vi "scanallvalues.vi"(0 "VISA resource name out":refnum<visa-resource-name>, 1 "nm ch":i32[](array[numeric]), 2 "Voltages values":dbl[](array[numeric]), 3 "Init clip value":i32[](array[numeric]), 4 "base path":path, 5 "error in":errorcluster, 6 "Integration Board IP":string, 7 "L1 Address":i32, 8 "Save test data":bool=TRUE, 9 "Ch burst":i32, 11 "Init att value":i32[](array[numeric])) -> (14 "50%":dbl[][][][](array[numeric]), 15 "L1 min values":i32[](array[numeric])=[180, 378, 779, 1613, 2478, 4286, 5228, 6743], 19 "error out":errorcluster)   [LabVIEW 2009]
uses:
  <instrlib>/Agilent 81150/Agilent 81150.lvlib
  <vilib>/Analysis/NI_AALPro.lvlib
panel:
  out "Data out":string="ACK\r\n"
  out "XY Graph":cluster{"Y":dbl[], "Y":dbl[]}[](graph)
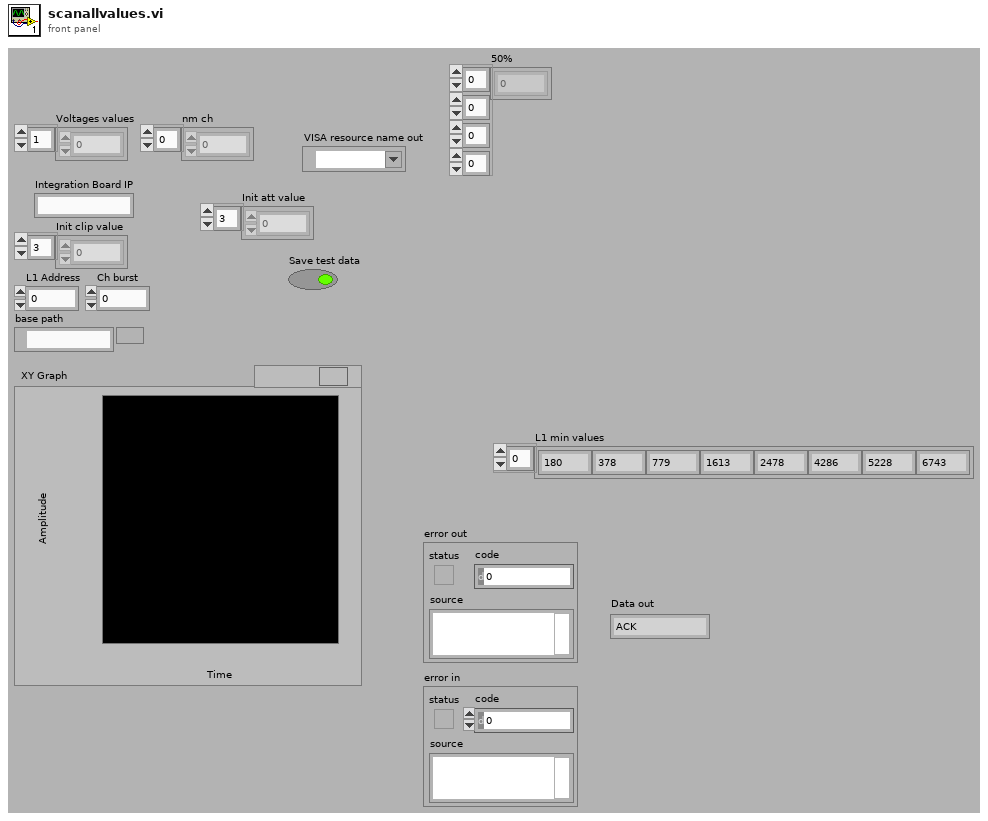
[diagram p1: front panel]
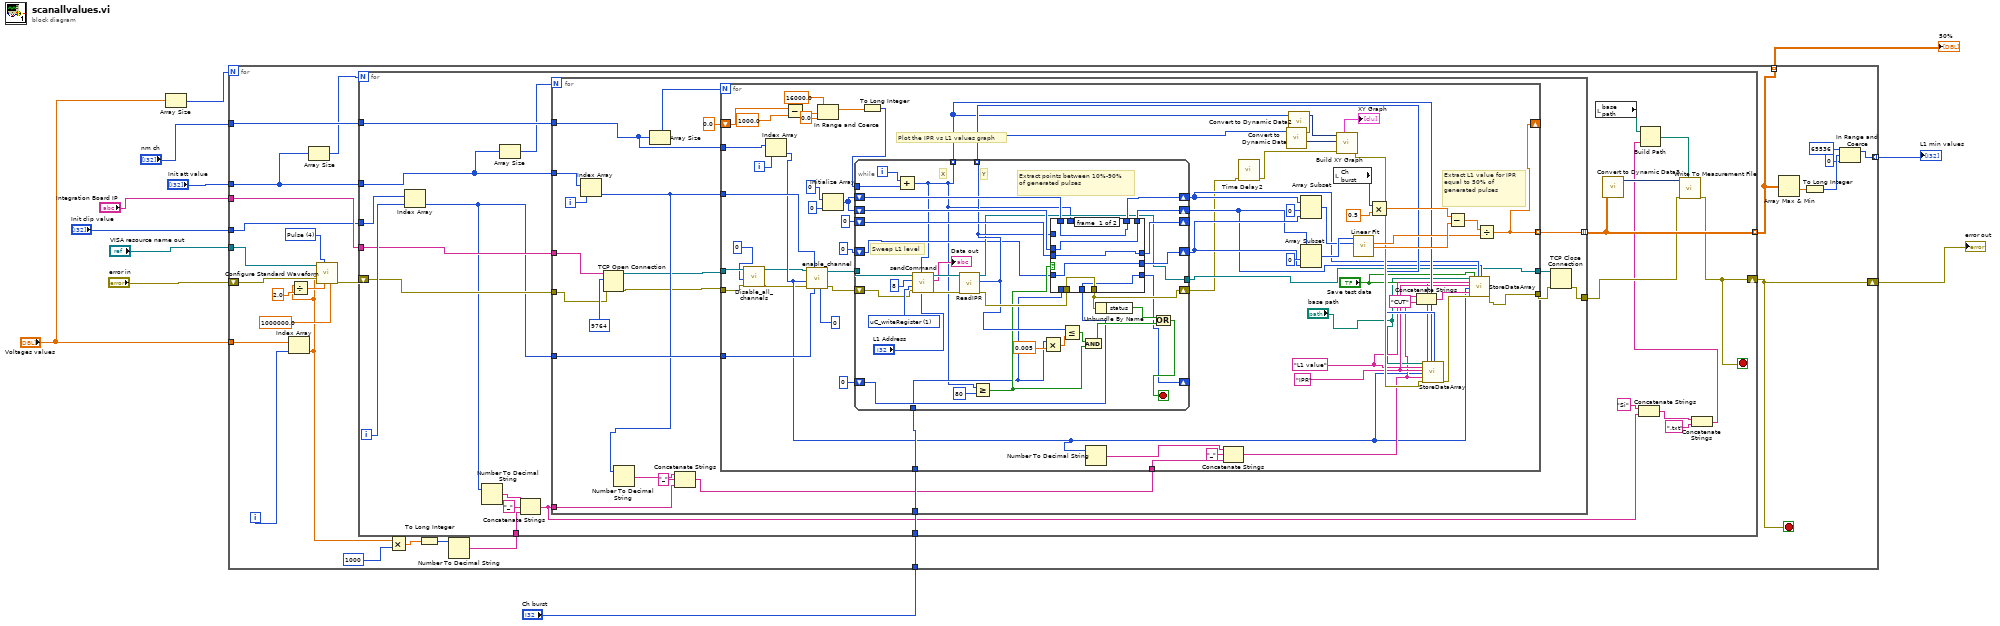
[diagram p0: block diagram]
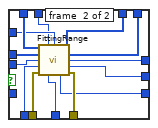
[diagram p2: hidden frame]
diagram:
  n1 = Array Size(array="Voltages values") -> (size(s)=w5:i32)
  n2 = for {
    N: w5 -> [_]
    shift-right: [w26] -> w11
    shift-left: "error in" -> [w25]
    tunnel: [w32] -> w10 mode=indexing
    tunnel: [w28] -> w1 mode=indexing
    tunnel: "Integration Board IP" -> [w27]
    tunnel: "VISA resource name out" -> [w29]
    tunnel: "Voltages values" -> [w19]
    tunnel: "Init clip value" -> [w18]
    tunnel: "Ch burst" -> [w17]
    tunnel: "nm ch" -> [w16]
    tunnel: "Init att value" -> [w14]
    i -> [w34]
    stop <- w26 stop-if-true
    w38 = u16 4 items=["Sine", "Square", "Ramp Up", "Ramp Down", "Pulse", "Noise", "DC"] ("Waveform (0: Sine)")
    n3 = Index Array(array=w19, index=w34) -> (element=w22:dbl)
    n4 = Divide(x=w22, y=2.0) -> (x/y=w36:dbl)
    n5 = Array Size(array=w14) -> (size(s)=w15:i32)
    n6 = call <instrlib>:"Configure Standard Waveform.vi"("Frequency (1000.0 Hz)"=1000000.0, "DC Offset (0.0 Volts)"=w36, "Waveform (0: Sine)"=w38, "error in (no error)"=w25, "Amplitude (1.0 Vpp)"=w22, "VISA resource name"=w29) -> ("error out"=w24:errorcluster)  [unwired: 4 in, 1 out]
    n7 = Multiply(x=w22, y=1000) -> (x*y=w21:dbl)
    n8 = To Long Integer(number=w21) -> (32bit integer=w20:i32)
    n9 = Number To Decimal String(number=w20) -> (decimal integer string=w13:string)  [unwired: 1 in]
    n10 = for {
      N: w15 -> [_]
      tunnel: [w54] -> w28 mode=indexing
      shift-right: [w51] -> w26
      shift-left: w24 -> [w58]
      tunnel: w27 -> [w59]
      tunnel: w18 -> [w61]
      tunnel: w17 -> [w60]
      tunnel: w16 -> [w57]
      tunnel: w14 -> [w56]
      tunnel: w13 -> [w48]
      i -> [w62]
      stop <- w51 stop-if-true
      n11 = Index Array(array=w61, index=w62) -> (element=w50:i32)
      n12 = Number To Decimal String(number=w50) -> (decimal integer string=w47:string)  [unwired: 1 in]
      n13 = Array Size(array=w56) -> (size(s)=w55:i32)
      n14 = Concatenate Strings(w47, "_" ("string"), w48) -> (w40:string)
      n15 = for {
        N: w55 -> [_]
        tunnel: [w83] -> w54 mode=indexing
        tunnel: w60 -> [w82]
        tunnel: [w67] -> w52
        tunnel: w59 -> [w80]
        tunnel: w58 -> [w79]
        tunnel: w57 -> [w75]
        tunnel: w56 -> [w78]
        tunnel: w50 -> [w74]
        tunnel: w40 -> [w72]
        i -> [w77]
        n16 = Index Array(array=w78, index=w77) -> (element=w73:i32)
        n17 = TCP Open Connection(address=w80, remote port or service name=u16 9764, error in (no error)=w79) -> (connection ID=w65:refnum<k5>, error out=w64:errorcluster)  [unwired: 2 in]
        n18 = Number To Decimal String(number=w73) -> (decimal integer string=w71:string)  [unwired: 1 in]
        n19 = Array Size(array=w75) -> (size(s)=w76:i32)
        n20 = Concatenate Strings(w71, "_" ("string"), w72) -> (w69:string)
        n21 = for {
          N: w76 -> [_]
          tunnel: [w91] -> w83 mode=indexing
          tunnel: w82 -> [w122]
          tunnel: [w119] -> w68
          tunnel: w64 -> [w95]
          tunnel: w65 -> [w94]
          tunnel: w73 -> [w107]
          tunnel: w75 -> [w106]
          tunnel: w74 -> [w104]
          tunnel: w69 -> [w103]
          tunnel: [w98] -> w66
          shift-right: [w91] -> _
          shift-left: 0.0 -> [w90]
          i -> [w105]
          w128 = "IPR" ("Y Signal Name")
          w129 = "L1 value" ("X Signal Name")
          # "Extract L1 value for IPR equal to 50% of generated pulses"
          # "Plot the IPR vs L1 values graph"
          n22 = call "Disable_all_channels.vi"("error in"=w95, "id_in"=0, "connection ID"=w94) -> ("error out"=w96:errorcluster, "connection ID out"=w93:refnum<k5>)  [unwired: 6 in, 1 out]
          n23 = Index Array(array=w106, index=w105) -> (element=w100:i32)
          n24 = Subtract(x=w90, y=1000.0) -> (x-y=w86:dbl)
          n25 = call "enable_channel.vi"("Delay"=0 ("V clip"), "V clip"=w104, "V att"=w107, "error in"=w96, "Channel"=w100, "connection ID"=w93) -> ("error out"=w110:errorcluster, "connection ID out"=w109:refnum<k5>)  [unwired: 3 in, 1 out]
          n26 = In Range and Coerce(upper limit=16000.0, x=w86, lower limit=0.0) -> (coerced(x)=w87:dbl)  [unwired: 1 out]
          n27 = Initialize Array(0 ("element"), 0 ("dimension size")) -> (w114:i32[])
          n28 = To Long Integer(number=w87) -> (32bit integer=w88:i32)
          n29 = while {
            tunnel: [w162] -> w131 mode=indexing
            tunnel: [w147] -> w130 mode=indexing
            shift-right: [w177] -> w127
            shift-left: w114 -> [w175]
            shift-right: [w176] -> w126
            shift-left: w114 -> [w174]
            shift-right: [w170] -> w97
            shift-left: w110 -> [w155]
            shift-right: [w172] -> _
            shift-left: 0 ("Array Pointer out") -> [w173]
            tunnel: w109 -> [w156]
            tunnel: [w157] -> w98
            shift-right: [w171] -> w140
            shift-left: 0 ("N_Array Elements") -> [w153]
            shift-right: [w151] -> _
            shift-left: 0 ("State machine") -> [w152]
            tunnel: w122 -> [w149]
            tunnel: w88 -> [w146]
            i -> [w148]
            stop <- w168 stop-if-true
            w166 = u16 1 items=["sendCommand"=9, "FPGA_writeRegister"=3, "FPGA_readRegister"=2, "uC_writeRegister"=1, "uC_readRegister"=0] ("Action")
            # "Extract points between 10%-90% of generated pulses"
            # "Sweep L1 level"
            # "Y"
            # "X"
            n30 = Add(x=w148, y=w146) -> (x+y=w147:i32)
            n31 = call "sendCommand.vi"("Address"="L1 Address", "Data"=w147, "error in"=w155, "Action"=w166, "id_in"=8 ("id"), "connection ID"=w156) -> ("error out"=w165:errorcluster, "Data out"=→"Data out":string, "connection ID out"=w164:refnum<k5>)  [unwired: 1 in, 2 out]
            n32 = call "ReadIPR.vi"("error in"=w165, "connection ID"=w164) -> ("error out"=w163:errorcluster, "IPR value"=w162:i32, "connection ID out"=w157:refnum<k5>)  [unwired: 7 in]
            n33 = Greater Or Equal?(x=w147, y=80) -> (x >= y?=w154:bool)
            n34 = Multiply(x=w149, y=0.005) -> (x*y=w178:dbl)
            n35 = case shown="True" w154 {
              tunnel: [w185 w199] -> w177
              tunnel: [w184 w198] -> w176
              tunnel: w175 -> [w185 w197]
              tunnel: w174 -> [w184 w196]
              tunnel: w173 -> [w182 w195]
              tunnel: [w182 w194] -> w172
              tunnel: [w181 w193] -> w171
              tunnel: w149 -> [_ w192]
              tunnel: [w183 w191] -> w170
              tunnel: w163 -> [w183 w190]
              tunnel: w162 -> [_ w189]
              tunnel: w147 -> [_ w188]
              tunnel: w153 -> [w181 _]
              tunnel: w152 -> [w180 w187]
              tunnel: [w180 w186] -> w151
              frame #0 {
              }
              frame #1 {
                n36 = call "FittingRange.vi"("Array in (X)"=w197, "L0 DAC"=w188, "IPR"=w189, "Array in (Y)"=w196, "Array Pointer in"=w195, "Cycles Burst"=w192, "error in"=w190, "State machine"=w187) -> ("Array out (X)"=w199:i32[], "Array out (Y)"=w198:i32[], "Array Pointer out"=w194:i32, "N_Array Elements"=w193:i32, "State machine"=w186:i32, "error out"=w191:errorcluster)  [unwired: 2 in]
              }
            }
            n37 = Less Or Equal?(x=w162, y=w178) -> (x <= y?=w161:bool)
            n38 = And(x=w161, y=w154) -> (x .and. y?=w160:bool)
            n39 = Unbundle By Name(w170) -> ("status"=w169:bool)
            n40 = Or(x=w169, y=w160) -> (x .or. y?=w168:bool)
          }
          n41 = Number To Decimal String(number=w100) -> (decimal integer string=w99:string)  [unwired: 1 in]
          n42 = Concatenate Strings(w99, "_" ("string"), w103) -> (w102:string)
          n43 = call "Time Delay2"("error in (no error)"=w97) -> ("error out"=w118:errorcluster)  [unwired: 10 in]
          n44 = call "Convert to Dynamic Data"("Array"=w131) -> ("Dynamic Data Type"=w144:dynamicdata)  [unwired: 3 in]
          n45 = call "Convert to Dynamic Data2"("Array"=w130) -> ("Dynamic Data Type"=w143:dynamicdata)  [unwired: 3 in]
          n46 = Array Subset(array=w126, index=0, length=w140) -> (w139:i32[])
          n47 = Array Subset(array=w127, index=0, length=w140) -> (w138:i32[])
          n48 = local read "Ch burst"() -> (w121:i32)
          n49 = call "Build XY Graph"("error in (no error)"=w118, "Y Input"=w144, "X Input"=w143) -> ("error out"=w132:errorcluster, "XY Graph"=→"XY Graph":cluster{"Y":dbl[], "Y":dbl[]}[])  [unwired: 7 in]
          n50 = call <vilib>:"Linear Fit.vi"("Y"=w139, "X"=w138) -> ("slope"=w133:dbl, "intercept"=w135:dbl)  [unwired: 9 in, 3 out]
          n51 = Multiply(x=w121, y=0.5) -> (x*y=w136:dbl)
          n52 = Concatenate Strings(w102, "CUT" ("string")) -> (w124:string)
          n53 = call "StoreDataArray.vi"("Base path"="base path", "X Signal Name"=w129, "Y Signal Name"=w128, "Channel number"=w100, "Si"=w102, "error in"=w132, "Save test data"="Save test data", "X Array"=w130, "Y Array"=w131) -> ("error out"=w125:errorcluster)  [unwired: 10 in]
          n54 = Subtract(x=w136, y=w135) -> (x-y=w134:dbl)
          n55 = call "StoreDataArray.vi"("Base path"="base path", "X Signal Name"=w129, "Y Signal Name"=w128, "Channel number"=w100, "Si"=w124, "error in"=w125, "Save test data"="Save test data", "X Array"=w127, "Y Array"=w126) -> ("error out"=w119:errorcluster)  [unwired: 10 in]
          n56 = Divide(x=w134, y=w133) -> (x/y=w91:dbl)
        }
        n57 = TCP Close Connection(connection ID=w66, error in (no error)=w68) -> (error out=w67:errorcluster)  [unwired: 1 in, 1 out]
      }
      n58 = local read "base path"() -> (w46:path)
      n59 = call "Convert to Dynamic Data3"("2D Array"=w54) -> ("Dynamic Data Type"=w53:dynamicdata)  [unwired: 3 in]
      n60 = Concatenate Strings("Si" ("string"), w40) -> (w42:string)
      n61 = Concatenate Strings(w42, ".txt" ("string")) -> (w41:string)
      n62 = Build Path(base path=w46, name or relative path=w41) -> (appended path=w45:path)
      n63 = call "Write To Measurement File"("Signals"=w53, "error in (no error)"=w52, "Filename"=w45) -> ("error out"=w51:errorcluster)  [unwired: 14 in, 2 out]
    }
    n64 = Array Max & Min(array=w28) -> (min value=w35:dbl)  [unwired: 3 out]
    n65 = To Long Integer(number=w35) -> (32bit integer=w33:i32)
    n66 = In Range and Coerce(upper limit=65536, x=w33, lower limit=0) -> (coerced(x)=w32:i32)  [unwired: 1 out]
  }
  "L1 min values" <- w10
  "error out" <- w11
  "50%" <- w1
